vi "Add(SGL).vi"(1 "Enable(T)":bool=TRUE, 2 "In":sgl, 4 "n":sgl=1.0) -> (6 "Out":sgl=1.0 format="%.2f")   [LabVIEW 2013]
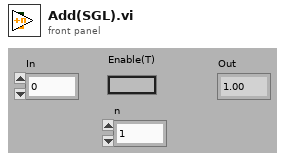
[diagram p1: front panel]
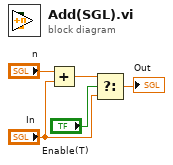
[diagram p0: block diagram]
diagram:
  n1 = Add(x="n", y="In") -> (x+y=w1:sgl)
  n2 = Select(t=w1, s="Enable(T)", f="In") -> (s? t:f=→"Out":sgl)
